vi "Error Calculation.vi"(10 "Dataset":T2, 11 "Predictions":sgl[][](array[numeric])) -> (3 "Depth":T1, 5 "MAE":dbl, 7 "MSE":dbl)   [LabVIEW 2020]
uses:
  <vilib>/Ngene/DeepLTK/Toolkit/NN_Data/API/DataSet_Types/NN_DataSet(In3D_Out1D).ctl
  <vilib>/Ngene/DeepLTK/Toolkit/NN_Data/API/DataRef_Types/NN_Data_ref(4D_SGL).ctl
  <vilib>/Ngene/DeepLTK/Toolkit/NN_Data/API/DataRef_Types/NN_Data_ref(2D_SGL).ctl
  <vilib>/Ngene/DeepLTK/Toolkit/NN_Data/API/DataRef_Types/NN_Data_ref(1D_I32).ctl
  <vilib>/Ngene/DeepLTK/Toolkit/NN_Data/Controls/NN_Dims(C,H,W).ctl
  Controls/FittingReport.ctl
  <vilib>/Analysis/baseanly.llb/Mean (DBL).vi
  <vilib>/Ngene/DeepLTK/Toolkit/NN_Data/subVIs/Get_Data_Vals/NN_Data_Get_ValByRef(2D_SGL).vi
  <vilib>/Analysis/NI_AALBase.lvlib
  <vilib>/Ngene/DeepLTK/Toolkit/Deep_Learning_Toolkit_by_Ngene.lvlib
panel:
  out "GT vs Pred (Depth)":sgl[][](graph)
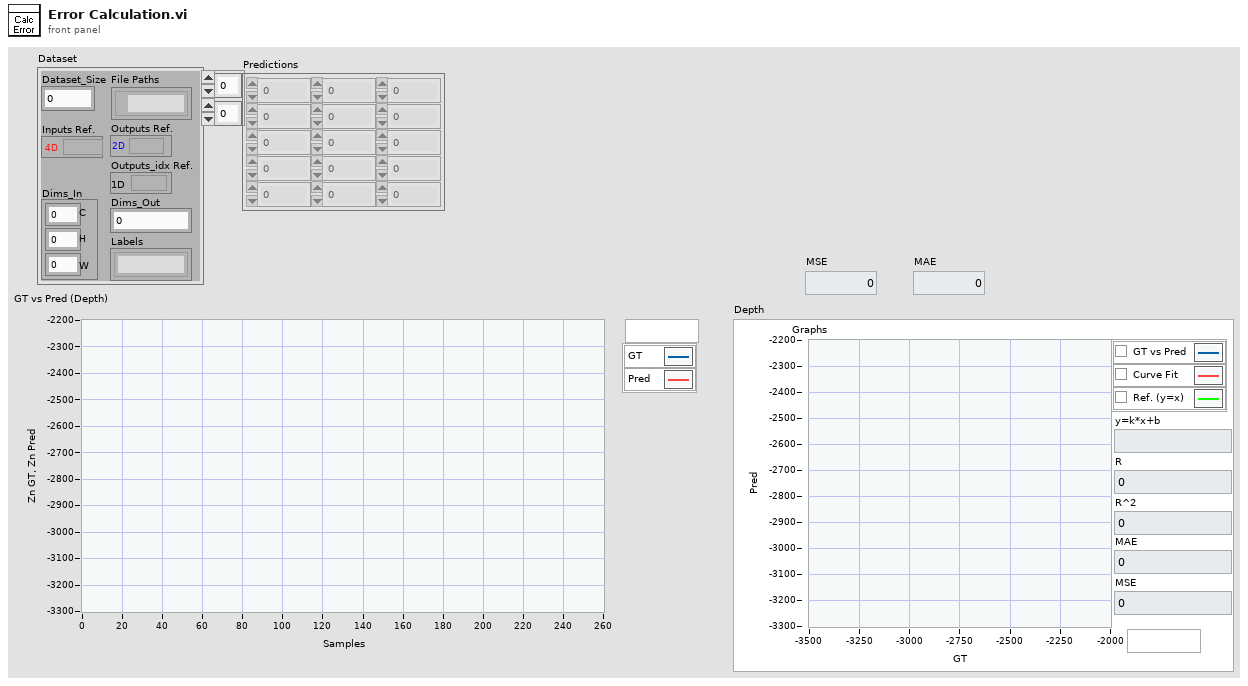
[diagram p1: front panel]
types:
  T1 = typedef "FittingReport.ctl" = cluster{"Graphs":cluster{"Best Linear Fit":dbl[], "Array 3":sgl[]}[], "y=k*x+b":string, "R":sgl, "R^2":sgl, "MAE":sgl, "MSE":sgl}
  T2 = typedef "Deep_Learning_Toolkit_by_Ngene.lvlib/NN_DataSet(In3D_Out1D).ctl" = cluster{"Inputs Ref.":T3, "Outputs Ref.":T4, "Dataset_Size":i32, "Outputs_idx Ref.":T5, "Dims_In":T6, "Dims_Out":i32, "Labels":string[], "File Paths":path[]}
  T3 = typedef "Deep_Learning_Toolkit_by_Ngene.lvlib/NN_Data_ref(4D_SGL).ctl" = refnum<data-value>
  T4 = typedef "Deep_Learning_Toolkit_by_Ngene.lvlib/NN_Data_ref(2D_SGL).ctl" = refnum<data-value>
  T5 = typedef "Deep_Learning_Toolkit_by_Ngene.lvlib/NN_Data_ref(1D_I32).ctl" = refnum<data-value>
  T6 = typedef "Deep_Learning_Toolkit_by_Ngene.lvlib/NN_Dims(C,H,W).ctl" = cluster{"C":i32, "H":i32, "W":i32}
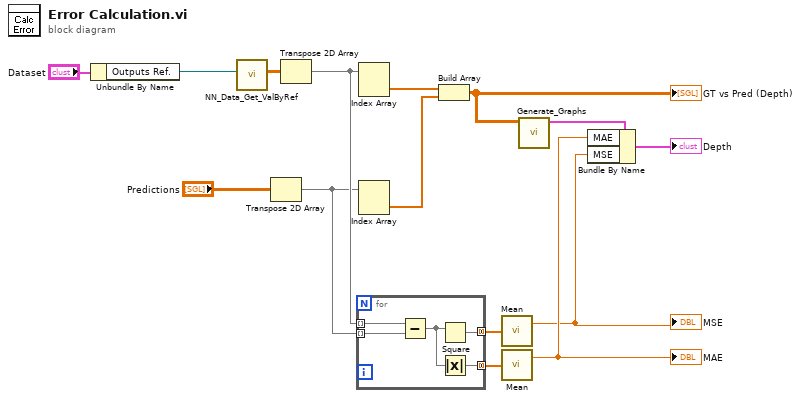
[diagram p0: block diagram]
diagram:
  n1 = Unbundle By Name("Dataset") -> ("Outputs Ref."=w9:T4)
  n2 = call-poly <vilib>:"NN_Data_Get_ValByRef.vi"("DVR(2D_SGL)"=w9) -> ("Value(2D_SGL)"=w8:sgl[][])  [unwired: 7 in, 1 out]
  n3 = Transpose 2D Array(2D array="Predictions") -> (transposed array=w10:sgl[][])
  n4 = Transpose 2D Array(2D array=w8) -> (transposed array=w11:sgl[][])
  n5 = for {
    tunnel: w11 -> [w17] mode=indexing
    tunnel: w10 -> [w16] mode=indexing
    tunnel: [w20] -> w13 mode=concatenating
    tunnel: [w18] -> w12 mode=concatenating
    n6 = Subtract(x=w17, y=w16) -> (x-y=w19:sgl[])
    n7 = Square(x=w19) -> (x^2=w20:sgl[])
    n8 = Absolute Value(x=w19) -> (abs(x)=w18:sgl[])
  }
  n9 = Index Array(array=w11) -> (element=w7:sgl[])  [unwired: 2 in]
  n10 = Index Array(array=w10) -> (element=w6:sgl[])  [unwired: 2 in]
  n11 = Build Array(w7, w6) -> (w5:sgl[][])
  "GT vs Pred (Depth)" <- w5
  n12 = call-poly <vilib>:"Mean.vi"("X"=w13) -> ("mean"=w1:dbl)  [unwired: 1 out]
  "MSE" <- w1
  n13 = call-poly <vilib>:"Mean.vi"("X"=w12) -> ("mean"=w2:dbl)  [unwired: 1 out]
  "MAE" <- w2
  n14 = call "Generate_Graphs.vi"("Data (GT, Pred)"=w5) -> ("Report"=w4:T1)  [unwired: 10 in]
  n15 = Bundle By Name(cluster=w4, "MAE"=w2, "MSE"=w1) -> (→"Depth":T1)
